vi "Move merged.vi"(6 "left":bool=TRUE, 7 "left exp":bool=TRUE, 8 "error in (no error)":errorcluster, 9 "vertical":bool=TRUE, 10 "pixel move":i32=1, 11 "Control-Client in":refnum<class "Control-Client.lvclass">) -> (0 "error out":errorcluster, 3 "Control-Client out":refnum<class "Control-Client.lvclass">)   [LabVIEW 2020, in "Control-Client.lvclass"]
uses:
  Control-Client.lvclass
  Experiments/Experiment_merged/Experiment_merged.lvclass
  C:/dev/TRANCON/Classes/Experiments/Experiment.lvclass
  Control-Client.lvclass/Control-Client.ctl
  Experiments/Experiment.lvclass
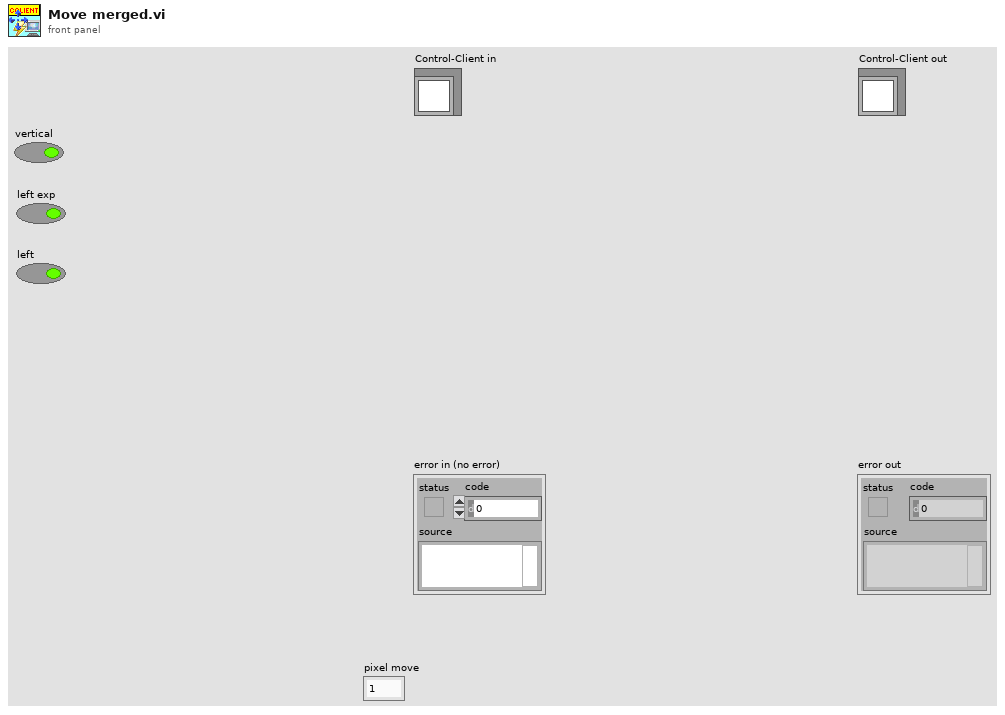
[diagram p1: front panel]
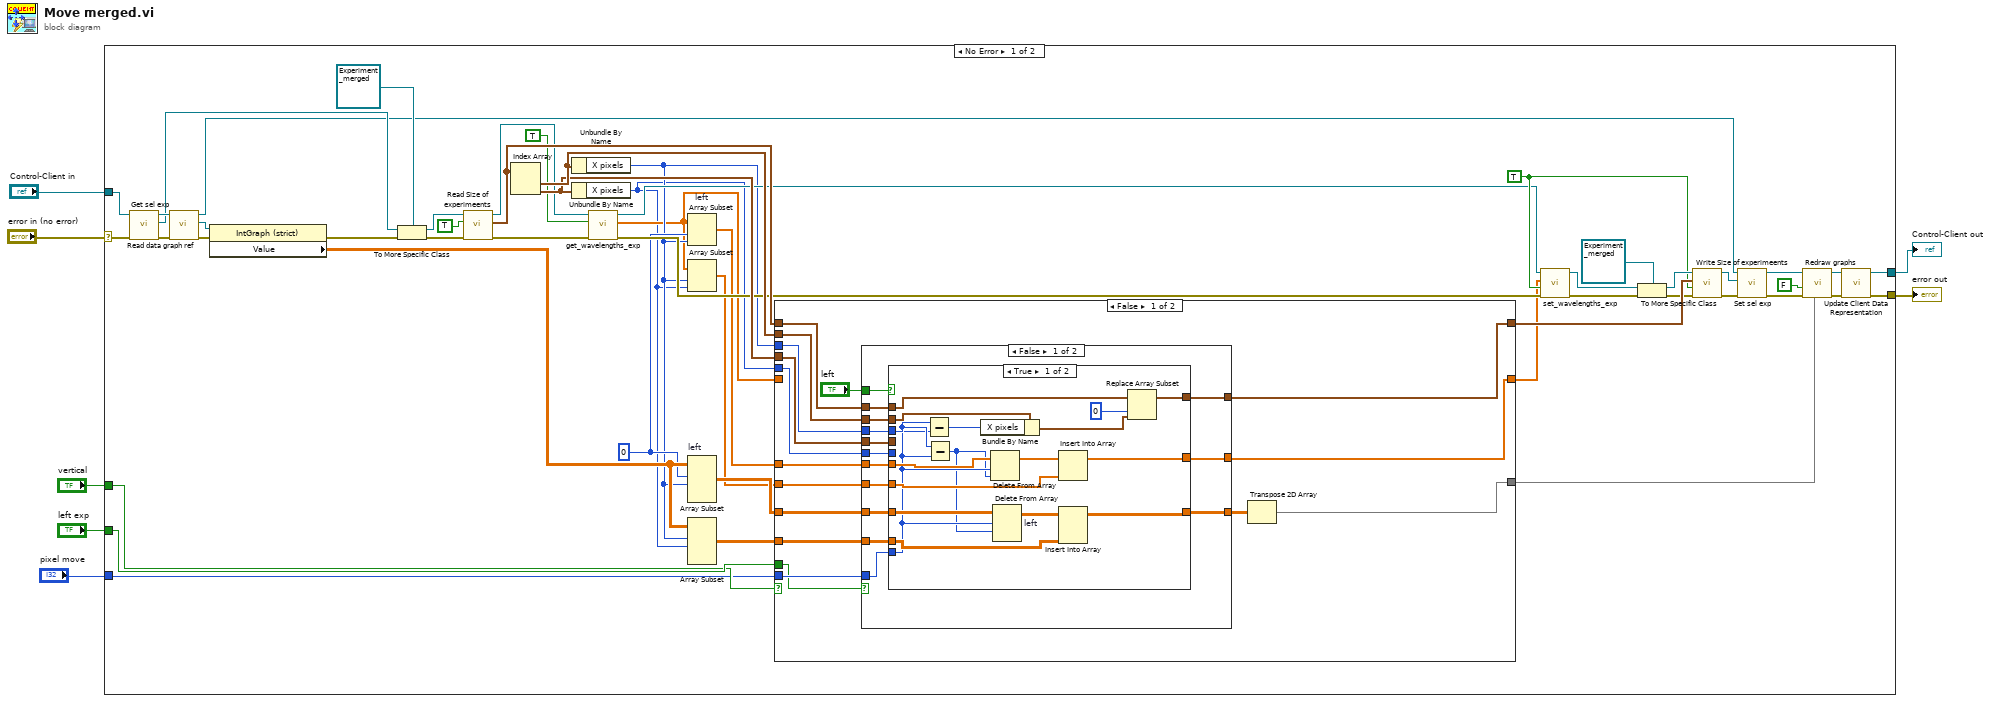
[diagram p0: block diagram]
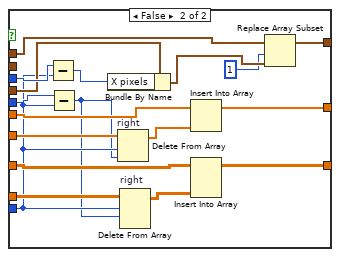
[diagram p2: hidden frame]
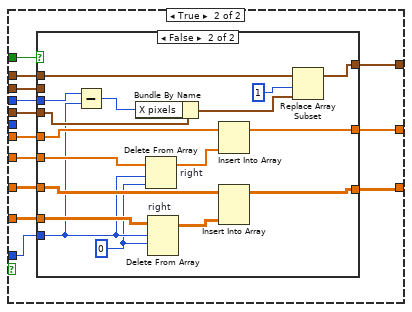
[diagram p3: hidden frame]
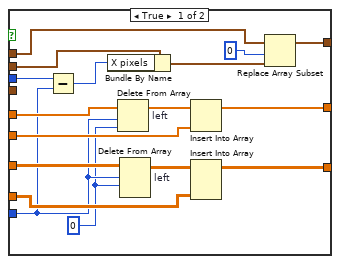
[diagram p4: hidden frame]
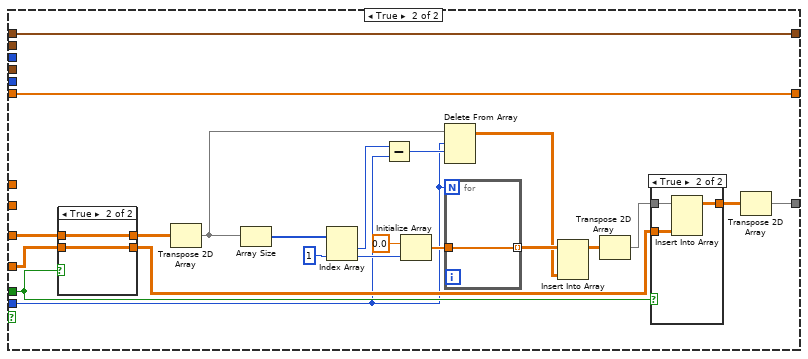
[diagram p5: hidden frame]
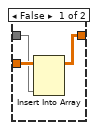
[diagram p6: hidden frame]
diagram:
  n1 = case shown="No Error" "error in (no error)" {
    selector: "error in (no error)" -> [w58 w205]
    tunnel: [w55 w205] -> w6
    tunnel: [w57 w204] -> w4
    tunnel: "Control-Client in" -> [w56 w204]
    tunnel: "pixel move" -> [w49 _]
    tunnel: "left exp" -> [w51 _]
    tunnel: "vertical" -> [w50 _]
    frame No Error {
      w19 = TRUE ("Temp")
      w13 = 0 ("index")
      n2 = call "Get sel exp.vi"("error in (no error)"=w58, "Control-Client in"=w56) -> ("error out"=w47:errorcluster, "Sel experiment"=w41:refnum<class "Experiment.lvclass">, "Control-Client out"=w46:refnum<class "Control-Client.lvclass">)  [unwired: 7 in]
      n3 = call "Read data graph ref.vi"("error in (no error)"=w47, "Control-Client in"=w46) -> ("error out"=w43:errorcluster, "Exp data graph ref"=w45:refnum<vi>, "Control-Client out"=w34:refnum<class "Control-Client.lvclass">)  [unwired: 7 in]
      n4 = property class="IntGraph (strict)"(reference=w45, error in=w43) -> (error out=w42:errorcluster, "Value"=w44:dbl[][])  [unwired: 1 out]
      n5 = To More Specific Class(target class=refnum<class "Experiment_merged.lvclass"> refnum ("Experiment_merged in"), reference=w41, error in=w42) -> (specific class reference=w39:refnum<class "Experiment_merged.lvclass">, error out=w40:errorcluster)
      n6 = call-dynamic "Read Size of experimeents.vi"("error in (no error)"=w40, "Temp"=TRUE, "Experiment_merged in"=w39) -> ("error out"=w16:errorcluster, "Size of experimeents"=w28:cluster{"X pixels":i32, "Y pixels":i32}[], "Experiment_merged out"=w15:refnum<class "Experiment_merged.lvclass">)  [unwired: 6 in]
      n7 = Index Array(array=w28) -> (element #1=w27:cluster{"X pixels":i32, "Y pixels":i32}, element #2=w26:cluster{"X pixels":i32, "Y pixels":i32})  [unwired: 2 in]
      n8 = Unbundle By Name(w27) -> ("X pixels"=w11:i32)
      n9 = Unbundle By Name(w26) -> ("X pixels"=w9:i32)
      n10 = call "get_wavelengths_exp.vi"("error in (no error)"=w16, "Temp"=TRUE, "Experiment.lvclass in"=w15) -> ("error out"=w18:errorcluster, "wavelengths"=w10:dbl[], "Experiment.lvclass out"=w17:refnum<class "Experiment_merged.lvclass">)  [unwired: 6 in]
      n11 = Array Subset "left"(array=w10, index=w13, length=w11) -> (w12:dbl[])
      n12 = Array Subset(array=w10, index=w11, length=w9) -> (w8:dbl[])
      n13 = Array Subset "left"(array=w44, index (row)=w13, length (row)=w11) -> (w36:dbl[][])  [unwired: 2 in]
      n14 = Array Subset(array=w44, index (row)=w11, length (row)=w9) -> (w35:dbl[][])  [unwired: 2 in]
      n15 = case shown="False" w50 {
        tunnel: w51 -> [w63 w186]
        tunnel: w49 -> [w73 w175]
        tunnel: [w64 w182] -> w48
        tunnel: w11 -> [w71 _]
        tunnel: w36 -> [w74 w181]
        tunnel: w35 -> [w72 w180]
        tunnel: [w62 w179] -> w29
        tunnel: w28 -> [w70 w179]
        tunnel: w27 -> [w69 _]
        tunnel: w26 -> [w68 _]
        tunnel: w9 -> [w66 _]
        tunnel: [w59 w171] -> w14
        tunnel: w10 -> [_ w171]
        tunnel: w12 -> [w61 _]
        tunnel: w8 -> [w60 _]
        frame False {
          n16 = case shown="False" w63 {
            tunnel: w74 -> [w87 w136]
            tunnel: w73 -> [w84 w135]
            tunnel: w72 -> [w85 w134]
            tunnel: [w79 w133] -> w65
            tunnel: w71 -> [w86 w132]
            tunnel: w70 -> [w81 w131]
            tunnel: w69 -> [w82 w130]
            tunnel: [w80 w129] -> w62
            tunnel: w68 -> [w83 w128]
            tunnel: "left" -> [w88 w127]
            tunnel: w66 -> [w78 _]
            tunnel: w61 -> [w76 w126]
            tunnel: w60 -> [w75 w125]
            tunnel: [w77 w124] -> w59
            frame False {
              n17 = case shown="True" w88 {
                tunnel: w87 -> [w105 w114]
                tunnel: w84 -> [w91 w107]
                tunnel: w85 -> [w103 w115]
                tunnel: [w102 w123] -> w79
                tunnel: w86 -> [w95 w122]
                tunnel: w81 -> [w99 w120]
                tunnel: w82 -> [w101 _]
                tunnel: [w96 w117] -> w80
                tunnel: w83 -> [_ w116]
                tunnel: w78 -> [_ w112]
                tunnel: [w89 w111] -> w77
                tunnel: w76 -> [w94 w109]
                tunnel: w75 -> [w92 w108]
                frame True {
                  n18 = Subtract(x=w95, y=w91) -> (x-y=w100:i32)
                  n19 = Subtract(x=w95, y=w91) -> (x-y=w90:i32)
                  n20 = Bundle By Name(cluster=w101, "X pixels"=w100) -> (w98:cluster{"X pixels":i32, "Y pixels":i32})
                  n21 = Delete From Array(array=w94, length=w91, index=w90) -> (array with subset deleted=w93:dbl[])  [unwired: 1 out]
                  n22 = Delete From Array "left"(array=w105, length=w91, index (row)=w90) -> (array with subset deleted=w104:dbl[][])  [unwired: 1 in, 1 out]
                  n23 = Insert Into Array(array=w93, new element=w92) -> (w89:dbl[])  [unwired: 1 in]
                  n24 = Insert Into Array(array=w104, new element=w103) -> (w102:dbl[][])  [unwired: 2 in]
                  n25 = Replace Array Subset(array=w99, new element=w98, index=0) -> (w96:cluster{"X pixels":i32, "Y pixels":i32}[])
                }
                frame False {
                  n26 = Subtract(x=w122, y=w107) -> (x-y=w121:i32)
                  n27 = Subtract(x=w112, y=w107) -> (x-y=w106:i32)
                  n28 = Bundle By Name(cluster=w116, "X pixels"=w121) -> (w119:cluster{"X pixels":i32, "Y pixels":i32})
                  n29 = Delete From Array "right"(array=w108, length=w107, index=w106) -> (array with subset deleted=w110:dbl[])  [unwired: 1 out]
                  n30 = Delete From Array "right"(array=w115, length=w107, index (row)=w106) -> (array with subset deleted=w113:dbl[][])  [unwired: 1 in, 1 out]
                  n31 = Insert Into Array(array=w109, new element=w110) -> (w111:dbl[])  [unwired: 1 in]
                  n32 = Insert Into Array(array=w114, new element=w113) -> (w123:dbl[][])  [unwired: 2 in]
                  n33 = Replace Array Subset(array=w120, new element=w119, index=1) -> (w117:cluster{"X pixels":i32, "Y pixels":i32}[])
                }
              }
            }
            frame True {
              n34 = case shown="False" w127 {
                tunnel: w136 -> [w153 w161]
                tunnel: w135 -> [w140 w155]
                tunnel: w134 -> [w151 w162]
                tunnel: [w150 w170] -> w133
                tunnel: w132 -> [w149 w169]
                tunnel: w131 -> [w146 w167]
                tunnel: w130 -> [w148 _]
                tunnel: [w143 w164] -> w129
                tunnel: w128 -> [_ w163]
                tunnel: w126 -> [w141 w156]
                tunnel: w125 -> [w142 w158]
                tunnel: [w137 w159] -> w124
                frame True {
                  w139 = 0 ("index (row)")
                  n35 = Subtract(x=w149, y=w140) -> (x-y=w147:i32)
                  n36 = Bundle By Name(cluster=w148, "X pixels"=w147) -> (w145:cluster{"X pixels":i32, "Y pixels":i32})
                  n37 = Delete From Array "left"(array=w141, length=w140, index=w139) -> (array with subset deleted=w138:dbl[])  [unwired: 1 out]
                  n38 = Delete From Array "left"(array=w153, length=w140, index (row)=w139) -> (array with subset deleted=w152:dbl[][])  [unwired: 1 in, 1 out]
                  n39 = Insert Into Array(array=w138, new element=w142) -> (w137:dbl[])  [unwired: 1 in]
                  n40 = Insert Into Array(array=w152, new element=w151) -> (w150:dbl[][])  [unwired: 2 in]
                  n41 = Replace Array Subset(array=w146, new element=w145, index=0) -> (w143:cluster{"X pixels":i32, "Y pixels":i32}[])
                }
                frame False {
                  w154 = 0 ("index (row)")
                  n42 = Subtract(x=w169, y=w155) -> (x-y=w168:i32)
                  n43 = Bundle By Name(cluster=w163, "X pixels"=w168) -> (w166:cluster{"X pixels":i32, "Y pixels":i32})
                  n44 = Delete From Array "right"(array=w158, length=w155, index=w154) -> (array with subset deleted=w157:dbl[])  [unwired: 1 out]
                  n45 = Delete From Array "right"(array=w162, length=w155, index (row)=w154) -> (array with subset deleted=w160:dbl[][])  [unwired: 1 in, 1 out]
                  n46 = Insert Into Array(array=w156, new element=w157) -> (w159:dbl[])  [unwired: 1 in]
                  n47 = Insert Into Array(array=w161, new element=w160) -> (w170:dbl[][])  [unwired: 2 in]
                  n48 = Replace Array Subset(array=w167, new element=w166, index=1) -> (w164:cluster{"X pixels":i32, "Y pixels":i32}[])
                }
              }
            }
          }
          n49 = Transpose 2D Array(2D array=w65) -> (transposed array=w64:dbl[][])
        }
        frame True {
          n50 = case shown="True" w186 {
            tunnel: [w201 w203] -> w187
            tunnel: w181 -> [w200 w203]
            tunnel: w180 -> [w201 w202]
            tunnel: [w200 w202] -> w184
            frame False {
            }
            frame True {
            }
          }
          n51 = Transpose 2D Array(2D array=w187) -> (transposed array=w189:dbl[][])
          n52 = Array Size(array=w189) -> (size(s)=w192:i32[])
          n53 = Index Array(array=w192, index #2=1 ("index")) -> (element #1=w178:i32, element #2=w188:i32)  [unwired: 1 in]
          n54 = Subtract(x=w178, y=w175) -> (x-y=w177:i32)
          n55 = Initialize Array(0.0 ("element"), w188) -> (w176:dbl[])
          n56 = Delete From Array(array=w189, length=w175, index (row)=w177) -> (array with subset deleted=w173:dbl[][])  [unwired: 1 in, 1 out]
          n57 = for {
            N: w175 -> [_]
            tunnel: w176 -> [w193]
            tunnel: [w193] -> w174 mode=indexing
          }
          n58 = Insert Into Array(array=w174, new element=w173) -> (w172:dbl[][])  [unwired: 2 in]
          n59 = Transpose 2D Array(2D array=w172) -> (transposed array=w185:dbl[][])
          n60 = case shown="True" w186 {
            tunnel: w185 -> [w195 w199]
            tunnel: w184 -> [w196 w198]
            tunnel: [w194 w197] -> w183
            frame False {
              n61 = Insert Into Array(array=w196, new element=w195) -> (w194:dbl[][])  [unwired: 2 in]
            }
            frame True {
              n62 = Insert Into Array(array=w199, new element=w198) -> (w197:dbl[][])  [unwired: 2 in]
            }
          }
          n63 = Transpose 2D Array(2D array=w183) -> (transposed array=w182:dbl[][])
        }
      }
      n64 = call "set_wavelengths_exp.vi"("error in (no error)"=w18, "Temp"=w19, "wavelengths"=w14, "Experiment.lvclass in"=w17) -> ("error out"=w21:errorcluster, "Experiment.lvclass out"=w20:refnum<class "Experiment_merged.lvclass">)  [unwired: 6 in]
      n65 = To More Specific Class(target class=refnum<class "Experiment_merged.lvclass"> refnum ("Experiment_merged in"), reference=w20, error in=w21) -> (specific class reference=w24:refnum<class "Experiment_merged.lvclass">, error out=w23:errorcluster)
      n66 = call-dynamic "Write Size of experimeents.vi"("error in (no error)"=w23, "Temp"=w19, "Size of experimeents"=w29, "Experiment_merged in"=w24) -> ("error out"=w31:errorcluster, "Experiment_merged out"=w30:refnum<class "Experiment_merged.lvclass">)  [unwired: 6 in]
      n67 = call "Set sel exp.vi"("error in (no error)"=w31, "Experiment"=w30, "Control-Client in"=w34) -> ("error out"=w33:errorcluster, "Control-Client out"=w32:refnum<class "Control-Client.lvclass">)  [unwired: 7 in]
      n68 = call "Redraw graphs.vi"("Data"=w48, "error in (no error)"=w33, "Selected exp"=FALSE, "Control-Client in"=w32) -> ("error out"=w54:errorcluster, "Control-Client out"=w53:refnum<class "Control-Client.lvclass">)  [unwired: 6 in]
      n69 = call "Update Client Data Representation.vi"("error in (no error)"=w54, "Control-Client in"=w53) -> ("error out"=w55:errorcluster, "Control-Client out"=w57:refnum<class "Control-Client.lvclass">)  [unwired: 8 in]
    }
    frame Error {
    }
  }
  "error out" <- w6
  "Control-Client out" <- w4
